vi "VariantToText.vi"(8 "error in (no error)":errorcluster, 10 "Variant":variant, 11 "BlueTOMLSerializer in":refnum<class "BlueTOMLSerializer.lvclass">) -> (0 "error out":errorcluster, 2 "Serializable Text":string, 3 "BlueTOMLSerializer out":refnum<class "BlueTOMLSerializer.lvclass">)   [LabVIEW 2019, in "BlueTOMLSerializer.lvlib" / "BlueTOMLSerializer.lvclass"]
uses:
  BlueTOMLSerializer.lvclass
  BlueTOMLSerializer.lvlib
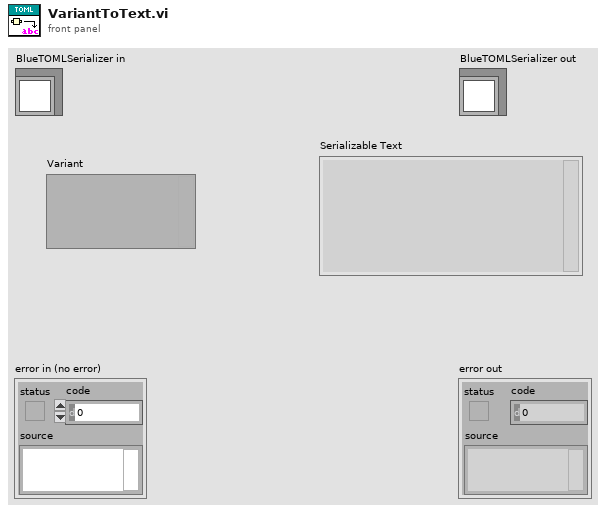
[diagram p1: front panel]
types:
  T1 = typedef "BlueTOMLSerializer.lvlib/TOML Value.ctl" = cluster{"\\type":enum16{"Table", "Array", "String", "Integer", "Float", "Boolean", "Offset Date-Time", "Local Date-Time", "Local Date", "Local Time"}, "ÿýÿýÿýÿýÿýÿþÿýÿýÿý%LV-TOML.lvlib:TOML Key-Value Pair.ctlÿýÿýÿýÿýÿýÿþÿýÿýÿýLV-TOML.lvlib:TOML Value.ctl$":variant}
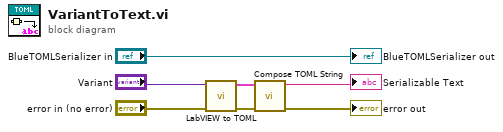
[diagram p0: block diagram]
diagram:
  n1 = call "LabVIEW to TOML.vi"("error in (no error)"="error in (no error)", "LV Value"="Variant") -> ("error out"=w6:errorcluster, "TOML Value"=w7:T1)  [unwired: 8 in]
  n2 = call "Compose TOML String.vi"("error in (no error)"=w6, "Value"=w7) -> ("error out"=→"error out":errorcluster, "String"=→"Serializable Text":string)  [unwired: 8 in]
  "BlueTOMLSerializer out" <- "BlueTOMLSerializer in"
